vi "Read (Multiple Digital Waveforms).vi"(8 "error in (no error)":errorcluster, 9 "Maximum Time (10000ms)":u32=10000, 10 "Digital Channels":u16[](array[ring])=[14] items=["Digital Channel D0"=14, "Digital Channel D1"=15, "Digital Channel D2"=16, "Digital Channel D3"=17, "Digital Channel D4"=18, "Digital Channel D5"=19, "Digital Channel D6"=20, "Digital Channel D7"=21, "Digital Channel D8"=22, "Digital Channel D9"=23, "Digital Channel D10"=24, "Digital Channel D11"=25, "Digital Channel D12"=26, "Digital Channel D13"=27, "Digital Channel D14"=28, "Digital Channel D15"=29], 11 "VISA resource name":refnum<visa-resource-name>) -> (0 "error out":errorcluster, 2 "Digital Waveform Graph":digitalwaveform[](graph), 3 "VISA resource name out":refnum<visa-resource-name>)   [LabVIEW 2009, in "Tektronix DPO MSO 2000 4000 Series.lvlib"]
doc: "Initiates an acquisition on all channels that you enabled with the <B>Configure Digital Channel</B> VI. The VI waits for the acquisition to complete and returns the waveform for the <B>Digital Channels</B> you specified. The <B>Maximum Time</B> control specifies the maximum time to wait for operation complete in milliseconds. If the oscilloscope did not complete the acquisition within the time period you specify with the <B>Maximum Time</B> parameter, the VI returns a timeout error. A common cause for a timeout error is the acquisition was not triggered. For example, the trigger level is out of range of the waveform. \n\n<B>Note:</B> LabVIEW versions higher than 7.1 might display the data differently."
uses:
  <instrlib>/Tektronix DPO MSO 2000 4000 Series/Tektronix DPO MSO 2000 4000 Series.lvlib
  <instrlib>/Tektronix DPO MSO 2000 4000 Series/Public/Data/Data_Low Level/Fetch Waveform (Digital Waveform).vi
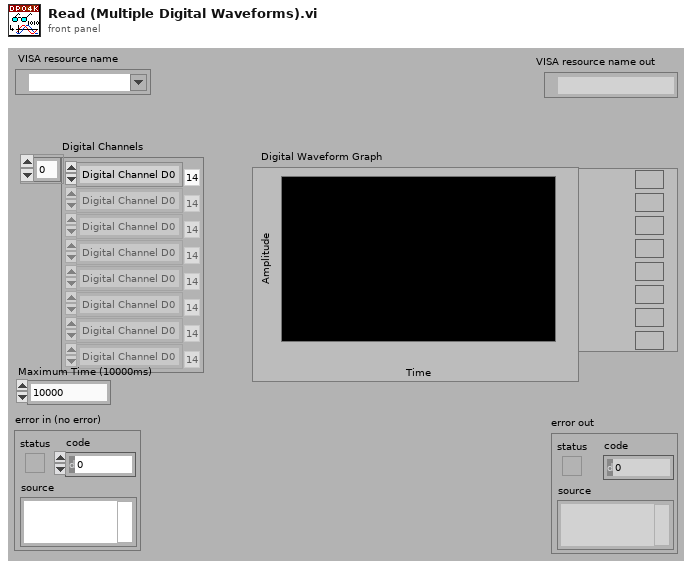
[diagram p1: front panel]
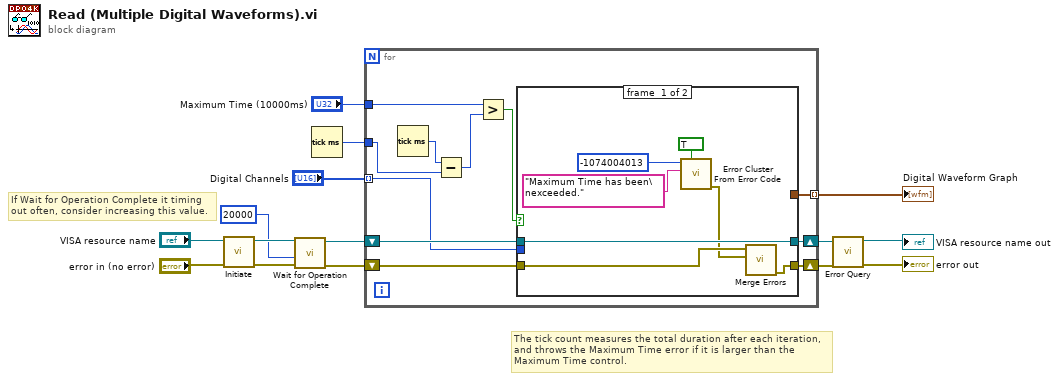
[diagram p0: block diagram]
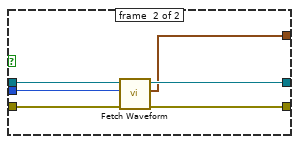
[diagram p2: hidden frame]
diagram:
  # "If Wait for Operation Complete it timing out often, consider increasing this value."
  # "The tick count measures the total duration after each iteration, and throws the Maximum Time error if it is larger than the Maximum Time control."
  n1 = call <instrlib>:"Initiate.vi"("error in (no error)"="error in (no error)", "VISA resource name"="VISA resource name") -> ("error out"=w7:errorcluster, "VISA resource name out"=w8:refnum<visa-resource-name>)  [unwired: 8 in]
  n2 = call <instrlib>:"Wait for Operation Complete.vi"("error in (no error)"=w7, "Maximum Time (10000ms)"=u32 20000, "VISA resource name"=w8) -> ("error out"=w5:errorcluster, "VISA resource name out"=w6:refnum<visa-resource-name>)  [unwired: 7 in]
  n3 = Tick Count (ms)() -> (millisecond timer value=w3:u32)
  n4 = for {
    shift-right: [w24] -> w14
    shift-left: w6 -> [w25]
    shift-right: [w23] -> w13
    shift-left: w5 -> [w26]
    tunnel: "Digital Channels" -> [w22] mode=indexing
    tunnel: w3 -> [w20]
    tunnel: "Maximum Time (10000ms)" -> [w19]
    tunnel: [w16] -> w1 mode=indexing
    n5 = Tick Count (ms)() -> (millisecond timer value=w21:u32)
    n6 = Subtract(x=w21, y=w20) -> (x-y=w18:u32)
    n7 = Greater?(x=w19, y=w18) -> (0:w17:bool)
    n8 = case shown="True" w17 {
      tunnel: w26 -> [w28 w39]
      tunnel: w25 -> [w33 w38]
      tunnel: [w33 w37] -> w24
      tunnel: [w29 w36] -> w23
      tunnel: w22 -> [_ w35]
      tunnel: [_ w34] -> w16
      frame #0 {
        n9 = call <vilib>:"Error Cluster From Error Code.vi"("show call chain? (False)"=TRUE, "error message (\"\")"="Maximum Time has been\nexceeded." ("error message (\"\")"), "error code (0)"=-1074004013) -> ("error out"=w27:errorcluster)  [unwired: 6 in]
        n10 = call <vilib>:"Merge Errors.vi"("error in 2 (no error)"=w27, "error in 1 (no error)"=w28) -> ("error out"=w29:errorcluster)  [unwired: 5 in]
      }
      frame #1 {
        n11 = call-poly <instrlib>:"Fetch Waveform.vi"("error in (no error)"=w39, "Digital Channel (14: Digital Channel D0)"=w35, "VISA resource name"=w38) -> ("error out"=w36:errorcluster, "Digital Waveform"=w34:digitalwaveform, "VISA resource name out"=w37:refnum<visa-resource-name>)  [unwired: 6 in]
      }
    }
  }
  "Digital Waveform Graph" <- w1
  n12 = call <instrlib>:"Error Query.vi"("error in (no error)"=w13, "VISA resource name"=w14) -> ("error out"=→"error out":errorcluster, "VISA resource name out"=→"VISA resource name out":refnum<visa-resource-name>)  [unwired: 6 in, 2 out]
